vi "Get-Set NLLM Fit Status.vi"(0 "Fit Parameters":dbl[](array[numeric]), 1 "chiSqr":dbl, 2 "Lambda":dbl, 4 "Get(F)/Set":bool, 5 "Error In":errorcluster, 6 "NL Fit Method":T2, 7 "|Delta Chi 2|/Chi 2":dbl, 8 "# Iterations":i32, 9 "Max |Delta a| /|a|":dbl, 10 "# Function Calls":i32, 11 "|Delta Chi 2|":dbl, 13 "Done":bool) -> (14 "NLLM Status":T1, 19 "Error Out":errorcluster)   [LabVIEW 2021, in "Fits.lvlib"]
uses:
  Fits.lvlib
  Nonlinear Fit Method.ctl
  Non-linear Fit Status Data.ctl
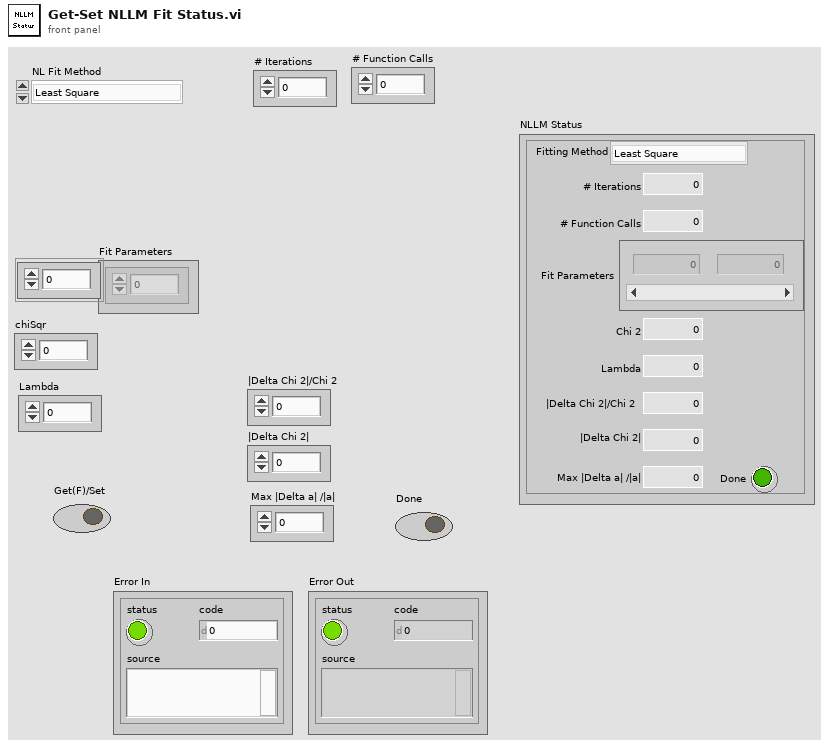
[diagram p1: front panel]
types:
  T1 = typedef "Fits.lvlib/Non-linear Fit Status Data.ctl" = cluster{"Fitting Method":T2, "# Iterations":i32, "# Function Calls":i32, "Fit Parameters":dbl[], "Chi 2":dbl, "Lambda":dbl, "|Delta Chi 2|/Chi 2":dbl, "|Delta Chi 2|":dbl, "Max |Delta a| /|a|":dbl, "Done":bool}
  T2 = typedef "Fits.lvlib/Nonlinear Fit Method.ctl" = enum16{"Least Square", "Least Absolute Residual", "Bisquare", "MLE"}
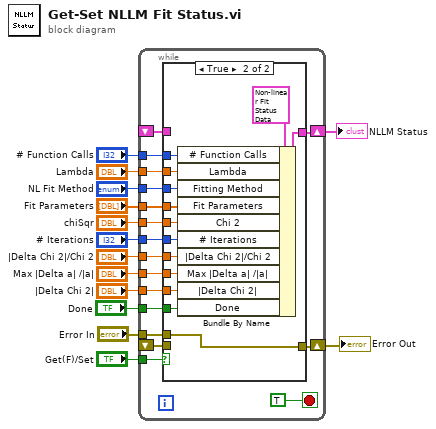
[diagram p0: block diagram]
diagram:
  n1 = while {
    tunnel: "Get(F)/Set" -> [w31]
    shift-right: [w20] -> w13
    shift-left: _ -> [w19]
    tunnel: "# Function Calls" -> [w29]
    tunnel: "NL Fit Method" -> [w28]
    tunnel: "Lambda" -> [w27]
    tunnel: "Fit Parameters" -> [w26]
    tunnel: "chiSqr" -> [w25]
    tunnel: "# Iterations" -> [w24]
    tunnel: "|Delta Chi 2|/Chi 2" -> [w23]
    tunnel: "Max |Delta a| /|a|" -> [w22]
    tunnel: "|Delta Chi 2|" -> [w21]
    tunnel: "Error In" -> [w18]
    shift-right: [w17] -> w2
    shift-left: _ -> [w16]
    tunnel: "Done" -> [w15]
    stop <- TRUE stop-if-true
    n2 = case shown="True" w31 {
      tunnel: w29 -> [_ w45]
      tunnel: w28 -> [_ w44]
      tunnel: w27 -> [_ w43]
      tunnel: w26 -> [_ w42]
      tunnel: w25 -> [_ w41]
      tunnel: w24 -> [_ w40]
      tunnel: w23 -> [_ w39]
      tunnel: w22 -> [_ w38]
      tunnel: w21 -> [_ w37]
      tunnel: [w33 w36] -> w20
      tunnel: w19 -> [w33 _]
      tunnel: w18 -> [_ w35]
      tunnel: [w32 w35] -> w17
      tunnel: w16 -> [w32 _]
      tunnel: w15 -> [_ w34]
      frame False {
      }
      frame True {
        n3 = Bundle By Name(cluster=T1 {"Fitting Method"=enum."Least Absolute Residual", "# Iterations"=0, "# Function Calls"=0, "Fit Parameters"=[], "Chi 2"=0.0, "Lambda"=0.0, "|Delta Chi 2|/Chi 2"=0.0, "|Delta Chi 2|"=0.0, "Max |Delta a| /|a|"=0.0, "Done"=FALSE} ("NLLM Status"), "# Function Calls"=w45, "Lambda"=w43, "Fitting Method"=w44, "Fit Parameters"=w42, "Chi 2"=w41, "# Iterations"=w40, "|Delta Chi 2|/Chi 2"=w39, "Max |Delta a| /|a|"=w38, "|Delta Chi 2|"=w37, "Done"=w34) -> (w36:T1)
      }
    }
  }
  "NLLM Status" <- w13
  "Error Out" <- w2
